vi "서브VI연습 (SubVI).vi"(6 "숫자형 4":dbl, 9 "숫자형 3":dbl, 10 "숫자형 입력":dbl, 11 "숫자형 5":dbl) -> (3 "숫자형 출력":dbl)   [LabVIEW 2020]
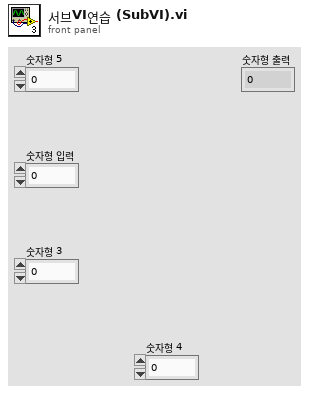
[diagram p1: front panel]
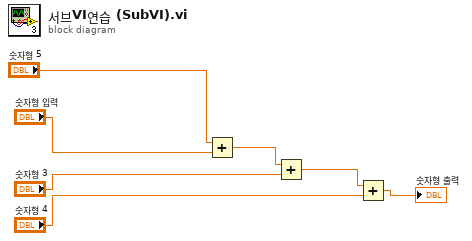
[diagram p0: block diagram]
diagram:
  n1 = Add(x="숫자형 5", y="숫자형 입력") -> (x+y=w3:dbl)
  n2 = Add(x=w3, y="숫자형 3") -> (x+y=w6:dbl)
  n3 = Add(x=w6, y="숫자형 4") -> (x+y=→"숫자형 출력":dbl)
